vi "HRM-Stage4-Process_main.vi"(8 "error in (no error)":errorcluster, 11 "Init cluster":T1) -> (0 "error out":errorcluster)   [LabVIEW 2020]
uses:
  HRM-Stage4-init_cluster.ctl
  HRM-Stage4-User_events.ctl
  <vilib>/measure/matone.llb/Extract Single Tone Information 1 Chan.vi
  <vilib>/measure/NI_MAPro.lvlib
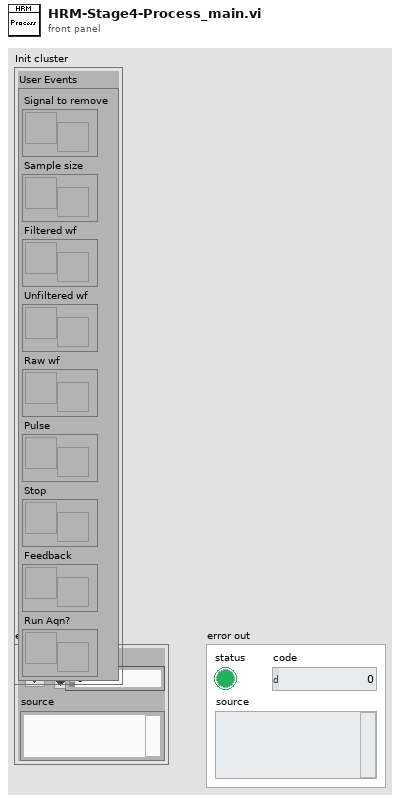
[diagram p1: front panel]
types:
  T1 = typedef "HRM-Stage4-init_cluster.ctl" = cluster{"User Events":T2}
  T2 = typedef "HRM-Stage4-User_events.ctl" = cluster{"Signal to remove":refnum<user-event>, "Sample size":refnum<user-event>, "Filtered wf":refnum<user-event>, "Unfiltered wf":refnum<user-event>, "Raw wf":refnum<user-event>, "Pulse":refnum<user-event>, "Stop":refnum<user-event>, "Feedback":refnum<user-event>, "Run Aqn?":refnum<user-event>}
  T3 = cluster{"Samples size (10)":i32, "Addition signal to remove":dbl, "Unfiltered wf":waveform(dbl), "User Events":T2}
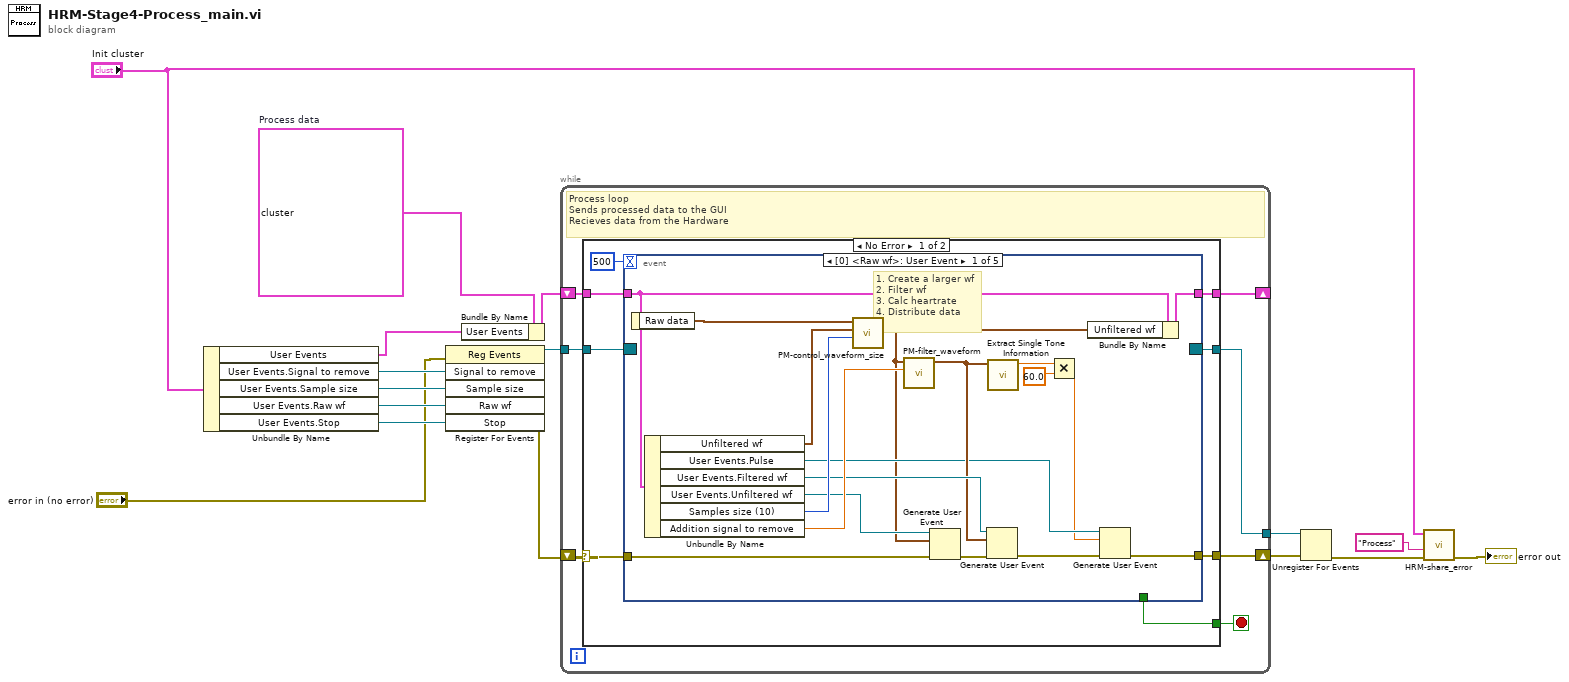
[diagram p0: block diagram]
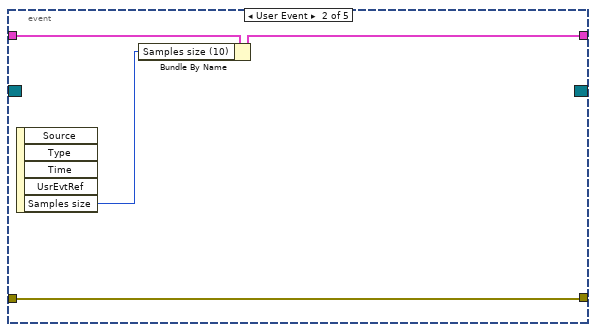
[diagram p2: hidden frame]
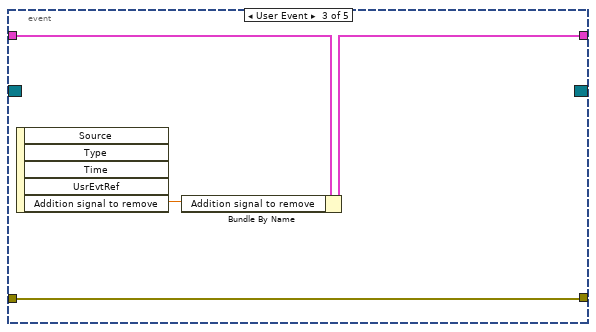
[diagram p3: hidden frame]
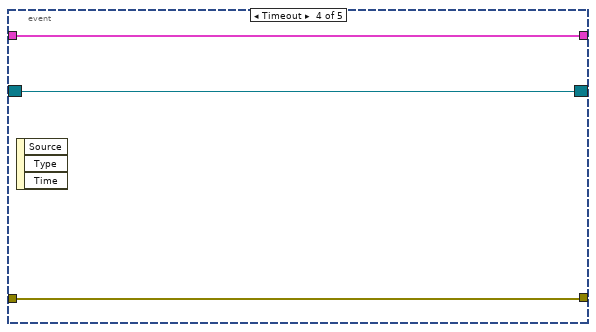
[diagram p4: hidden frame]
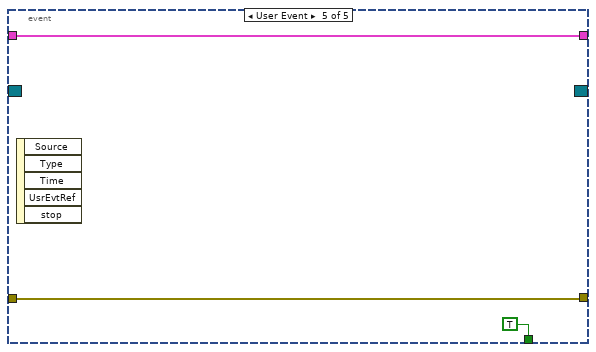
[diagram p5: hidden frame]
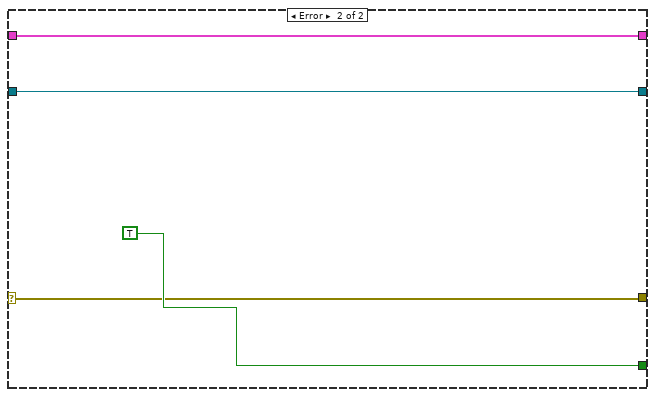
[diagram p6: hidden frame]
diagram:
  w7 = T3 {"Samples size (10)"=10, "Addition signal to remove"=0.0, "Unfiltered wf"={"t0"=timestamp(0 s since 1904-01-01), "dt"=1.0, "Y"=[]}, "User Events"={"Signal to remove"=refnum, "Sample size"=refnum, "Filtered wf"=refnum, "Unfiltered wf"=refnum, "Raw wf"=refnum, "Pulse"=refnum, "Stop"=refnum, "Feedback"=refnum, "Run Aqn?"=refnum}}  # Process data
  n1 = Unbundle By Name("Init cluster") -> ("User Events"=w16:T2, "User Events.Signal to remove"=w14:refnum<user-event>, "User Events.Sample size"=w13:refnum<user-event>, "User Events.Raw wf"=w12:refnum<user-event>, "User Events.Stop"=w15:refnum<user-event>)
  n2 = register-events(error in="error in (no error)", w14, w13, w12, w15) -> (reference out=w6:refnum<event-registration>, error out=w5:errorcluster)  [unwired: 1 in]
  n3 = Bundle By Name(cluster=w7, "User Events"=w16) -> (w8:T3)
  n4 = while {
    tunnel: w6 -> [w21]
    shift-right: [w19] -> _
    shift-left: w8 -> [w20]
    shift-right: [w18] -> w9
    shift-left: w5 -> [w22]
    tunnel: [w17] -> w10
    stop <- w23 stop-if-true
    # "Process loop\nSends processed data to the GUI\nRecieves data from the Hardware"
    n5 = case shown="No Error" w22 {
      selector: w22 -> [w28 w65]
      tunnel: [w24 TRUE ("Stop")] -> w23
      tunnel: w21 -> [w31 w64]
      tunnel: w20 -> [w30 w66]
      tunnel: [w29 w66] -> w19
      tunnel: [w27 w65] -> w18
      tunnel: [w25 w64] -> w17
      frame No Error {
        n6 = event shown="[0] <Raw wf>: User Event" {
          selector: w31 -> [_ _ _ w59 _]
          dyn-events: [_ _ _ w59 _] -> w25
          timeout: 500 -> [_ _ _ _ _]
          tunnel: w30 -> [w47 w53 w57 w60 w63]
          tunnel: [w36 w52 w56 w60 w63] -> w29
          tunnel: w28 -> [w33 w50 w54 w58 w61]
          tunnel: [w32 w50 w54 w58 w61] -> w27
          tunnel: [_ _ _ _ TRUE ("Stop")] -> w24
          event User Event {
            # "1. Create a larger wf\n2. Filter wf\n3. Calc heartrate\n4. Distribute data"
            n7 = event-data() -> ("Raw data"=w48:waveform(dbl))  [unwired: 1 in]
            n8 = Unbundle By Name(w47) -> ("Unfiltered wf"=w34:waveform(dbl), "User Events.Pulse"=w39:refnum<user-event>, "User Events.Filtered wf"=w42:refnum<user-event>, "User Events.Unfiltered wf"=w44:refnum<user-event>, "Samples size (10)"=w46:i32, "Addition signal to remove"=w45:dbl)
            n9 = call "PM-control_waveform_size.vi"("Samples s"=w46, "old waveform"=w34, "New waveform"=w48) -> ("waveform"=w35:waveform(dbl))  [unwired: 8 in]
            n10 = call "PM-filter_waveform.vi"("Addition signal to remove (0) [s]"=w45, "waveform in"=w35) -> ("waveform out"=w41:waveform(dbl))  [unwired: 8 in, 1 out]
            n11 = Generate User Event(user event=w44, event data cluster=w35, error in=w33) -> (error out=w43:errorcluster)  [unwired: 1 in, 1 out]
            n12 = Generate User Event(user event=w42, event data cluster=w41, error in=w43) -> (error out=w40:errorcluster)  [unwired: 1 in, 1 out]
            n13 = call-poly <vilib>:"Extract Single Tone Information.vi"("time signal in"=w41) -> ("detected frequency"=w38:dbl)  [unwired: 5 in, 5 out]
            n14 = Multiply(x=w38, y=60.0) -> (x*y=w37:dbl)
            n15 = Bundle By Name(cluster=w47, "Unfiltered wf"=w35) -> (w36:T3)
            n16 = Generate User Event(user event=w39, event data cluster=w37, error in=w40) -> (error out=w32:errorcluster)  [unwired: 1 in, 1 out]
          }
          event User Event {
            n17 = event-data() -> ("Samples size"=w51:i32)  [unwired: 1 in, 4 out]
            n18 = Bundle By Name(cluster=w53, "Samples size (10)"=w51) -> (w52:T3)
          }
          event User Event {
            n19 = event-data() -> ("Addition signal to remove"=w55:dbl)  [unwired: 1 in, 4 out]
            n20 = Bundle By Name(cluster=w57, "Addition signal to remove"=w55) -> (w56:T3)
          }
          event Timeout {
            n21 = event-data() -> ()  [unwired: 1 in, 3 out]
          }
          event User Event {
            n22 = event-data() -> ()  [unwired: 1 in, 5 out]
          }
        }
      }
      frame Error {
      }
    }
  }
  n23 = Unregister For Events(event registration refnum=w10, error in=w9) -> (error out=w4:errorcluster)
  n24 = call "HRM-share_error.vi"("error in (no error)"=w4, "module name"="Process", "Init cluster"="Init cluster") -> ("error out"=→"error out":errorcluster)  [unwired: 8 in]
